vi "Acknowledgement_RC.vi"(8 "error in (no error)":errorcluster, 10 "Acknowledgement_RC":T1, 11 "Rack Controller in":refnum<class "Rack Controller.lvclass">) -> (0 "error out":errorcluster, 3 "Rack Controller out":refnum<class "Rack Controller.lvclass">)   [LabVIEW 2019, in "Rack Controller.lvclass"]
uses:
  Rack Controller.lvclass
  <vilib>/ActorFramework/Message Enqueuer/Message Enqueuer.lvclass
  Common/Controls/Acknowledgement.ctl
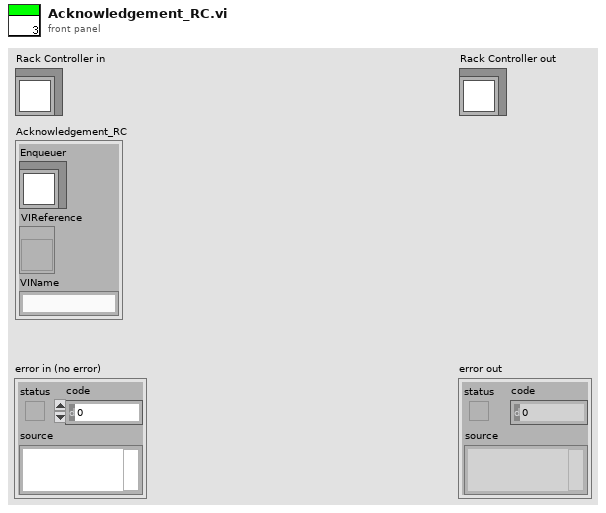
[diagram p1: front panel]
types:
  T1 = typedef "Acknowledgement.ctl" = cluster{"Enqueuer":refnum<class "Message Enqueuer.lvclass">, "VIReference":refnum<vi>, "VIName":string}
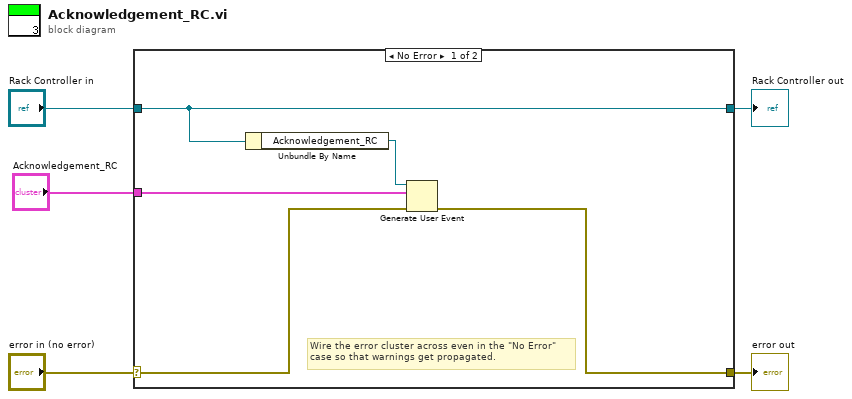
[diagram p0: block diagram]
diagram:
  n1 = case shown="No Error" "error in (no error)" {
    selector: "error in (no error)" -> [w7 w12]
    tunnel: [w6 w12] -> w4
    tunnel: [w9 w11] -> w2
    tunnel: "Rack Controller in" -> [w9 w11]
    tunnel: "Acknowledgement_RC" -> [w10 _]
    frame No Error {
      # "Wire the error cluster across even in the \"No Error\"\ncase so that warnings get propagated."
      n2 = Unbundle By Name(w9) -> ("Acknowledgement_RC"=w8:refnum<user-event>)
      n3 = Generate User Event(user event=w8, event data cluster=w10, error in=w7) -> (error out=w6:errorcluster)  [unwired: 1 in, 1 out]
    }
    frame Error {
    }
  }
  "error out" <- w4
  "Rack Controller out" <- w2
